vi "Create.vi"(8 "error in":errorcluster, 10 "reset":bool, 11 "option string":string) -> (0 "error out":errorcluster, 3 "Instrument out":refnum<class "Instrument.lvclass">)   [LabVIEW 2020, in "MeasurementLink niDCPower.lvlib" / "Instrument.lvclass"]
uses:
  Instrument.lvclass
  Instrument.lvclass/Instrument.ctl
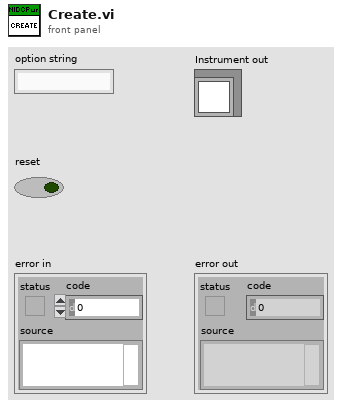
[diagram p1: front panel]
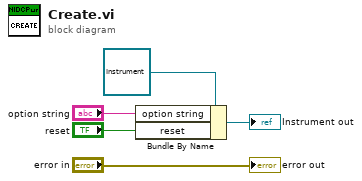
[diagram p0: block diagram]
diagram:
  n1 = Bundle By Name(cluster=refnum<class "Instrument.lvclass"> refnum ("Instrument in"), "option string"="option string", "reset"="reset") -> (→"Instrument out":refnum<class "Instrument.lvclass">)
  "error out" <- "error in"
